vi "verify_law.vi"() -> ()   [LabVIEW 2015]
panel:
  out "Boolean":bool
  in  "B":dbl
  in  "A":dbl
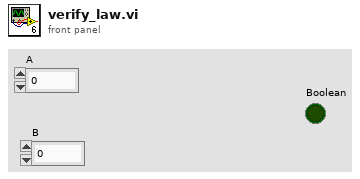
[diagram p1: front panel]
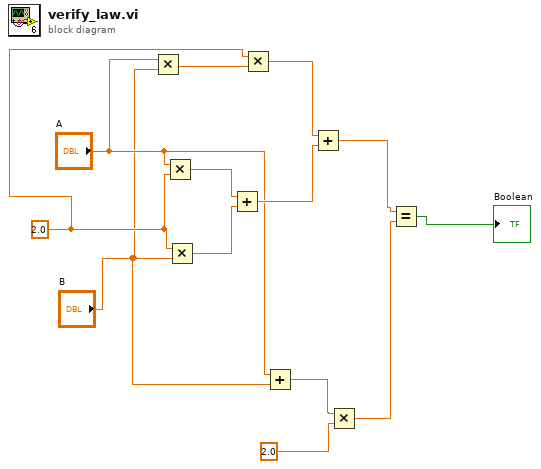
[diagram p0: block diagram]
diagram:
  w11 = 2.0 ("Numeric")
  n1 = Multiply(x="A", y="B") -> (x*y=w10:dbl)
  n2 = Multiply(x="A", y=w11) -> (x*y=w13:dbl)
  n3 = Multiply(x=w11, y="B") -> (x*y=w12:dbl)
  n4 = Add(x=w13, y=w12) -> (x+y=w9:dbl)
  n5 = Multiply(x=w11, y=w10) -> (x*y=w8:dbl)
  n6 = Add(x="A", y="B") -> (x+y=w4:dbl)
  n7 = Add(x=w8, y=w9) -> (x+y=w7:dbl)
  n8 = Multiply(x=w4, y=2.0 ("Numeric")) -> (x*y=w2:dbl)
  n9 = Equal?(x=w7, y=w2) -> (x = y?=→"Boolean":bool)
